vi "LVClass_ClosedLoopSecurityActivation_SetData.vi"(0 "ClosedLoopSecurity in":refnum<class "ClosedLoopSecurityActivation.lvclass">, 5 "ClosedLoopSecurityParams":T1, 11 "error in (no error)":errorcluster) -> (4 "ClosedLoopSecurity out":refnum<class "ClosedLoopSecurityActivation.lvclass">, 15 "error out":errorcluster)   [LabVIEW 2020, in "ClosedLoopSecurityActivation.lvclass"]
doc: "set switches states\n\n<B>security_activationIn</B> : Pointer to Closed Loop security activation object.\n<B>security_activationOut</B> : Pointer to Closed Loop security activation object.\n<B>do_check_saturated_act_count</B> : Activates the requested actuators positions check, test will return false if\n too many acturators reach their boundaries\n<B>do_check_camera_fill_pct</B> : Activates the camera saturation level check\n<B>do_check_pupil_size_variation</B> : Activates the pupil size variation check, test will return false if pupil is\n too different from the interaction matrix pupil\n<B>do_check_dwf_pv</B> : Activates the delta wavefront peak-to-valley check"
uses:
  ClosedLoopSecurityActivation.lvclass
  ClosedLoopSecurityActivationParameters.ctl
  ClosedLoopSecurityActivation.lvclass/ClosedLoopSecurityActivation.ctl
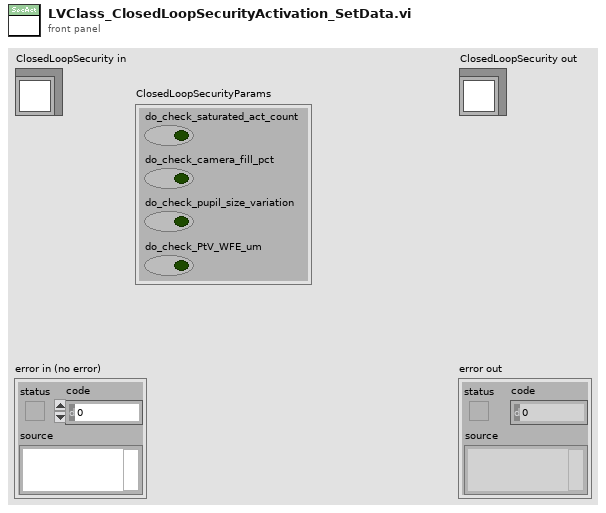
[diagram p1: front panel]
types:
  T1 = typedef "ClosedLoopSecurityActivationParameters.ctl" = cluster{"do_check_saturated_act_count":bool, "do_check_camera_fill_pct":bool, "do_check_pupil_size_variation":bool, "do_check_PtV_WFE_um":bool}
  T2 = typedef "ClassID.ctl" = i64
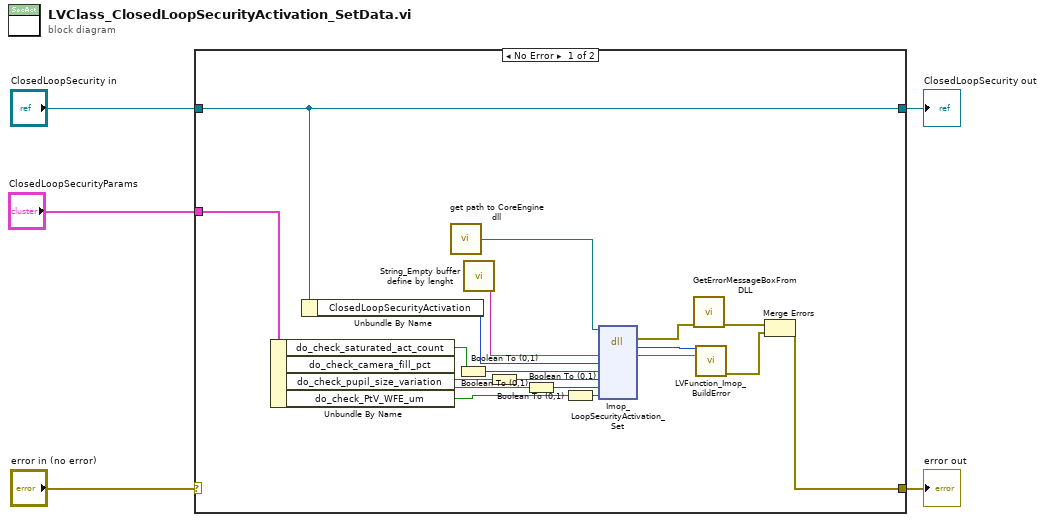
[diagram p0: block diagram]
diagram:
  n1 = case shown="No Error" "error in (no error)" {
    selector: "error in (no error)" -> [_ w26]
    tunnel: [w17 w26] -> w4
    tunnel: [w10 w25] -> w2
    tunnel: "ClosedLoopSecurity in" -> [w10 w25]
    tunnel: "ClosedLoopSecurityParams" -> [w16 _]
    frame No Error {
      n2 = Unbundle By Name(w16) -> ("do_check_saturated_act_count"=w15:bool, "do_check_camera_fill_pct"=w14:bool, "do_check_pupil_size_variation"=w13:bool, "do_check_PtV_WFE_um"=w12:bool)
      n3 = Unbundle By Name(w10) -> ("ClosedLoopSecurityActivation"=w11:T2)
      n4 = call "get path to CoreEngine dll.vi"() -> ("path to wavekit library"=w18:path)  [unwired: 14 in, 1 out]
      n5 = Boolean To (0,1)(Boolean=w15) -> (0, 1=w9:i16)
      n6 = call "String_Empty buffer define by lenght.vi"() -> ("Empty buffer"=w24:string)  [unwired: 1 in]
      n7 = Boolean To (0,1)(Boolean=w14) -> (0, 1=w8:i16)
      n8 = Boolean To (0,1)(Boolean=w13) -> (0, 1=w7:i16)
      n9 = Boolean To (0,1)(Boolean=w12) -> (0, 1=w6:i16)
      n10 = dll-call lib="D:/soft/HASO_v3/SVN_trunk/ImOpCoreEngine4_LV2011/DLLs/c_interface_vc100.dll" fn="Imop_LoopSecurityActivation_Set"(path in=w18, "message"=w24, "security_activation"=w11, "do_check_saturated_act_count"=w9, "do_check_camera_fill_pct"=w8, "do_check_pupil_size_variation"=w7, "do_check_loop_gain"=w6) -> (error out=w21:errorcluster, "return type"=w22:i32, "message"=w23:string)  [unwired: 7 in, 1 out]
      n11 = call "GetErrorMessageBoxFromDLL.vi"("error IN"=w21) -> ("error OUT"=w20:errorcluster)  [unwired: 10 in]
      n12 = call "LVFunction_Imop_BuildError.vi"("code"=w22, "String to Prepend to source (\"\")"=w23) -> ("error out"=w19:errorcluster)  [unwired: 13 in]
      n13 = Merge Errors(w20, w19) -> (w17:errorcluster)
    }
    frame Error {
    }
  }
  "error out" <- w4
  "ClosedLoopSecurity out" <- w2
